vi "Unflatten Value.vi"(8 "Error In":errorcluster, 10 "Value":string, 11 "2D Bool In":refnum<class "2D Bool.lvclass">) -> (0 "Error Out":errorcluster, 3 "2D Bool Out":refnum<class "2D Bool.lvclass">)   [LabVIEW 2020, in "NI_VIAnCFGDataStructure.lvlib" / "2D Bool.lvclass"]
doc: "Dynamic dispatch interface for unflattening Tree Data classes from string."
uses:
  <vilib>/addons/analyzer/VIAnCFGDataStructure/Data Types/2D Bool/2D Bool.lvclass
  <vilib>/addons/analyzer/VIAnCFGDataStructure/Data Types/2D Bool/2D Bool.lvclass/2D Bool.ctl
  <vilib>/addons/analyzer/VIAnCFGDataStructure/Tree Manager/Tree.lvclass
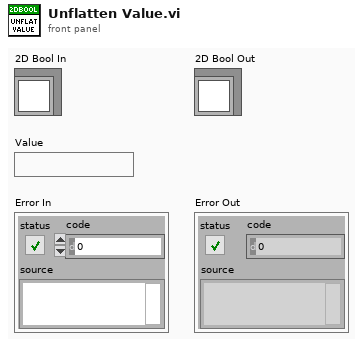
[diagram p1: front panel]
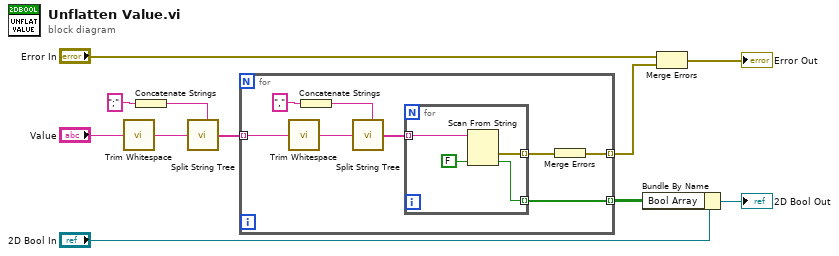
[diagram p0: block diagram]
diagram:
  n1 = call <vilib>:"Trim Whitespace.vi"("string"="Value") -> ("trimmed string"=w1:string)  [unwired: 1 in]
  n2 = Concatenate Strings(";" ("Separator (,)")) -> (w2:string)
  n3 = call <vilib>:"Split String Tree.vi"("Split Pattern"=w2, "Input String"=w1) -> ("Split String"=w11:string[])  [unwired: 5 in]
  n4 = for {
    tunnel: w11 -> [w18] mode=indexing
    tunnel: [w19] -> w7 mode=indexing
    tunnel: [w15] -> w5 mode=indexing
    n5 = call <vilib>:"Trim Whitespace.vi"("string"=w18) -> ("trimmed string"=w12:string)  [unwired: 1 in]
    n6 = Concatenate Strings("," ("Separator (,)")) -> (w13:string)
    n7 = call <vilib>:"Split String Tree.vi"("Split Pattern"=w13, "Input String"=w12) -> ("Split String"=w17:string[])  [unwired: 5 in]
    n8 = for {
      tunnel: w17 -> [w23] mode=indexing
      tunnel: [w21] -> w19 mode=indexing
      tunnel: [w20] -> w16 mode=indexing
      n9 = Scan From String(input string=w23, default 1=FALSE) -> (error out=w20:errorcluster, output 1=w21:bool)  [unwired: 3 in, 2 out]
    }
    n10 = Merge Errors(w16) -> (w15:errorcluster)
  }
  n11 = Bundle By Name(cluster="2D Bool In", "Bool Array"=w7) -> (→"2D Bool Out":refnum<class "2D Bool.lvclass">)
  n12 = Merge Errors("Error In", w5) -> (→"Error Out":errorcluster)
